vi "主程序-复材超声C扫缺陷分析评定软件.vi"() -> ()   [LabVIEW 2018]
doc: "使用该模板构建用户界面事件处理设计模式。将模板应用于对话框及其它用户界面。用户也可创建并执行VI可按照与用户界面事件相同方式处理的用户定义事件。"
uses:
  <vilib>/Utility/NIReport.llb/Report Type.ctl
  <vilib>/addons/_office/_exclsub.llb/font.ctl
  <vilib>/Utility/NIReport.llb/HTML Report Image Alignment.ctl
  <vilib>/Utility/NIReport.llb/Append Report Text (str wrap).vi
  <vilib>/Utility/NIReport.llb/Append Image to Report (path wrap).vi
  <vilib>/addons/_office/word.llb/Word Easy Table (str).vi
  <vilib>/Utility/NIReport.llb/NI_report.lvclass
  <vilib>/Utility/NIReport.llb/Word/NI_Word.lvclass
  <vilib>/addons/_office/NI_ReportGenerationToolkit.lvlib
  <vilib>/Utility/NIReport.llb/NI_ReportGenerationCore.lvlib
  <vilib>/vision/NI_Vision_Development_Module.lvlib
panel:
  out "是否需要预处理":u16
  out "数值":i8
  out "弥散类缺陷灰度阈值":dbl caption="值"
  out "计入分层缺陷的面积阈值":i32
  out "报告模式":string
  in  "删除标注":bool caption="定量分析"
  out "分层类缺陷灰度阈值":dbl caption="值"
  out "反射图原始路径":path
  out "穿透图原始路径":path
  out "ROImask":T1(plugin-control)
  out "模式选择":u16(ring) items=["只读穿透图", "穿透图和反射图结合"]
  out "添加的路径":path
  out "连接的字符串 2":string
  out "临界面积百分比值":dbl
  out "临界Z值":i32
  out "标注后的图片路径":path
  out "全部检测结果合并":string[][](table)
  out "全部检测结果":string[][](table)
  out "部位信息":string[](array[string])=["", "34.500000", "32.500000", "1121", "34", "54.955926", "分层类", "不合格", ""]
  out "连接的字符串":string
  in  "完成标注":bool caption="定量分析"
  out "框数":dbl
  out "自定义字体":T2={"Desired Font (Application)"=enum."Application Font", "[User-specified Font]"={"Font Name"="", "Size"=12, "Strikeout?"=FALSE, "Italic?"=FALSE, "Underline?"=FALSE, "Outline?"=FALSE, "Shadow?"=FALSE, "Bold?"=FALSE, "Rotation Angle"=0.0}, "Horizontal Alignment"=0, "Vertical Alignment"=0} {"Horizontal Alignment" items=["Left", "Center", "Right"]; "Vertical Alignment" items=["Bottom", "Top", "Baseline"]}
  out "框组":T3(array[cluster])
  out "质量等级":string
  in  "stop":bool caption="停止"
  in  "导入图像":bool caption="导入图片"
  in  "开始标注":bool caption="定量分析"
  in  "查看评定结果":bool caption="辅助定性分析"
  in  "生成报告":bool caption="生成原始记录"
  in  "控件":enum32{"穿透图", "反射图"}(tab)
  out "穿透图":T1(plugin-control)
  out "反射图":T1(plugin-control)
  out "产品规格":cluster{"产品长度（周长）（mm）":dbl, "产品宽度（母线长）（mm）":dbl}
  out "图像分辨率":T4
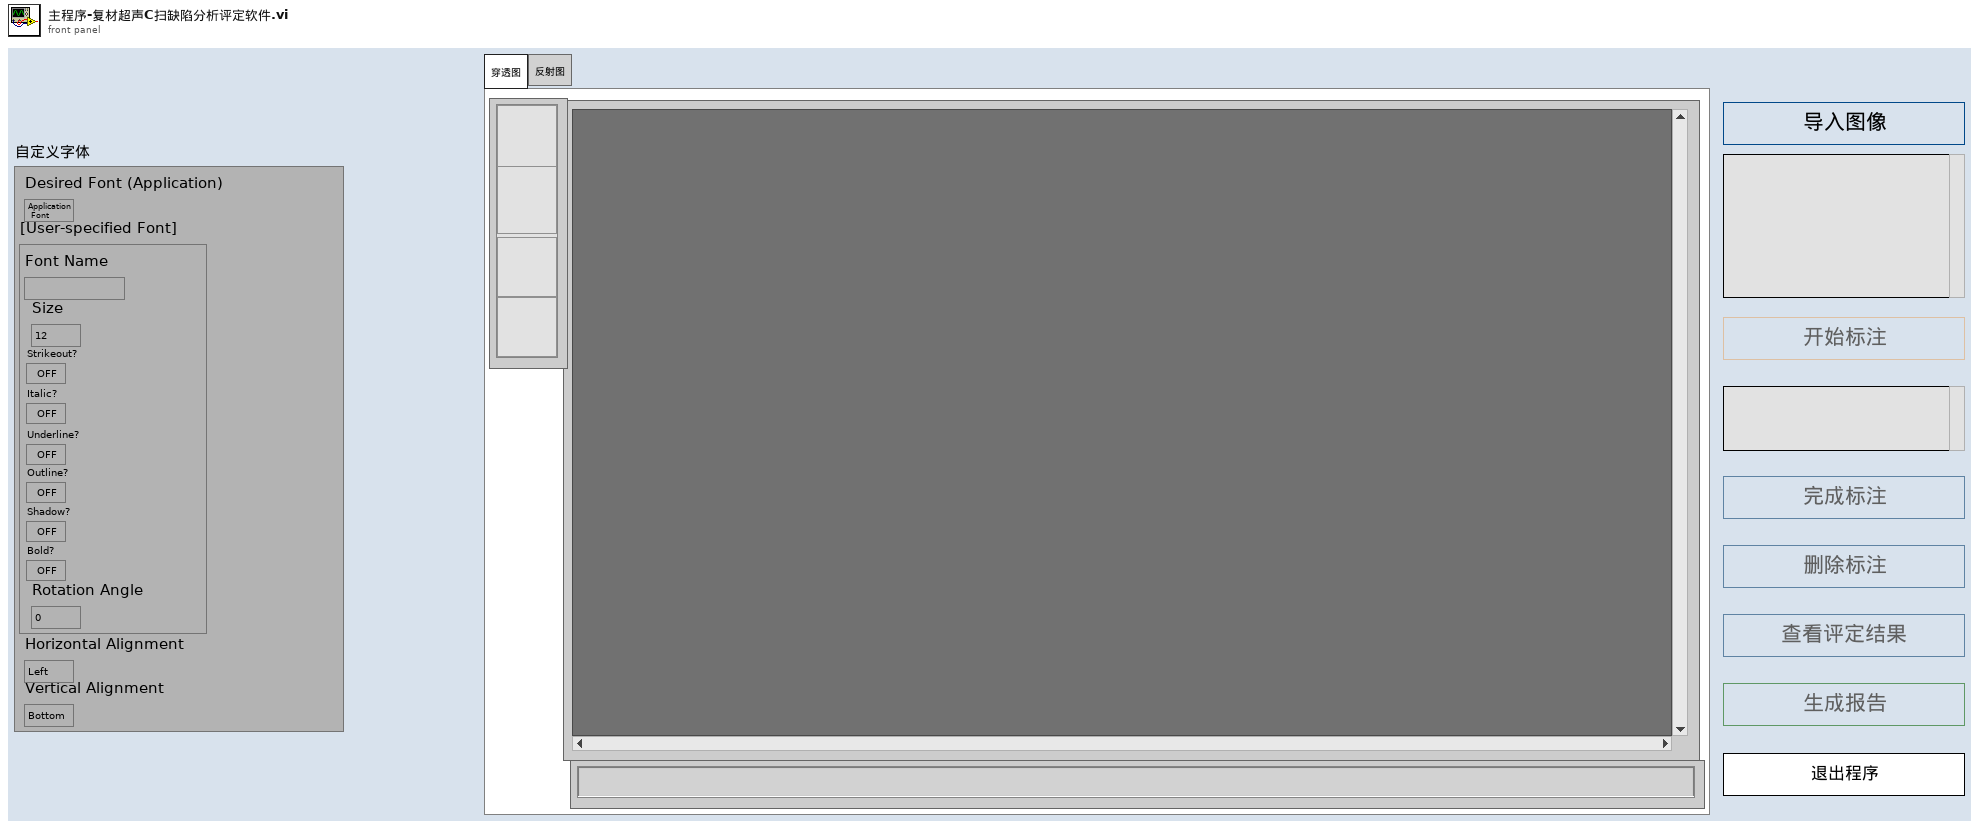
[diagram p1: front panel]
types:
  T1 = typedef "IMAQ Image.ctl" = refnum<image>
  T2 = cluster{"Desired Font (Application)":enum16{"User-specified Font", "Application Font", "System Font", "Dialog Font"}, "[User-specified Font]":cluster{"Font Name":string, "Size":i16, "Strikeout?":bool, "Italic?":bool, "Underline?":bool, "Outline?":bool, "Shadow?":bool, "Bold?":bool, "Rotation Angle":dbl}, "Horizontal Alignment":i16, "Vertical Alignment":i16}
  T3 = cluster{"Global Rectangle":i32[], "Contours":cluster{"Contour Type":u32, "ROI Type":u32, "Points":i32[]}[]}[]
  T4 = cluster{"图像X向分辨率（mm/像素）":dbl, "图像Y向分辨率（mm/像素）":dbl}
  T5 = enum8{"Enabled", "Disabled", "Disabled and Grayed Out"}
  T6 = cluster{"Global Rectangle":i32[], "Contours":cluster{"Contour Type":u32, "ROI Type":u32, "Points":i32[]}[]}
  T7 = cluster{"Zoom Tool":bool, "Selection Tool":bool, "Pan Tool":bool, "Point Tool":bool, "Line Tool":bool, "Rectangle Tool":bool, "Rotated Rectangle Tool":bool, "Polyline Tool":bool, "Polygon Tool":bool, "Freehand Tool":bool, "Closed Freehand Tool":bool, "Ellipse Tool":bool, "Annulus Tool":bool}
  T8 = enum16{"maximized", "minimized", "normal", "no change"}
  T9 = typedef "NI_ReportGenerationCore.lvlib/Report Type.ctl" = enum16{"HTML", "Word", "Excel"}
  T10 = typedef "NI_ReportGenerationCore.lvlib/HTML Report Image Alignment.ctl" = enum16{"(default)", "LEFT", "RIGHT", "TOP", "TEXTTOP", "MIDDLE", "ABSMIDDLE", "BASELINE", "BOTTOM", "ABSBOTTOM"}
  T11 = cluster{"position (Excel)":cluster{"row":i32, "column":i32}, "name (Excel)":string, "bookmark (Word)":string}
  T12 = cluster{"position (excel)":cluster{"row":i32, "column":i32}, "name (excel)":string, "bookmark (word)":string}
  T13 = typedef "NI_ReportGenerationToolkit.lvlib/font.ctl" = cluster{"font name":string, "font size":dbl, "bold":u16, "italic":u16, "underline":u16, "strike through":u16, "font color":u32}
  T14 = typedef "Image Type" = u32
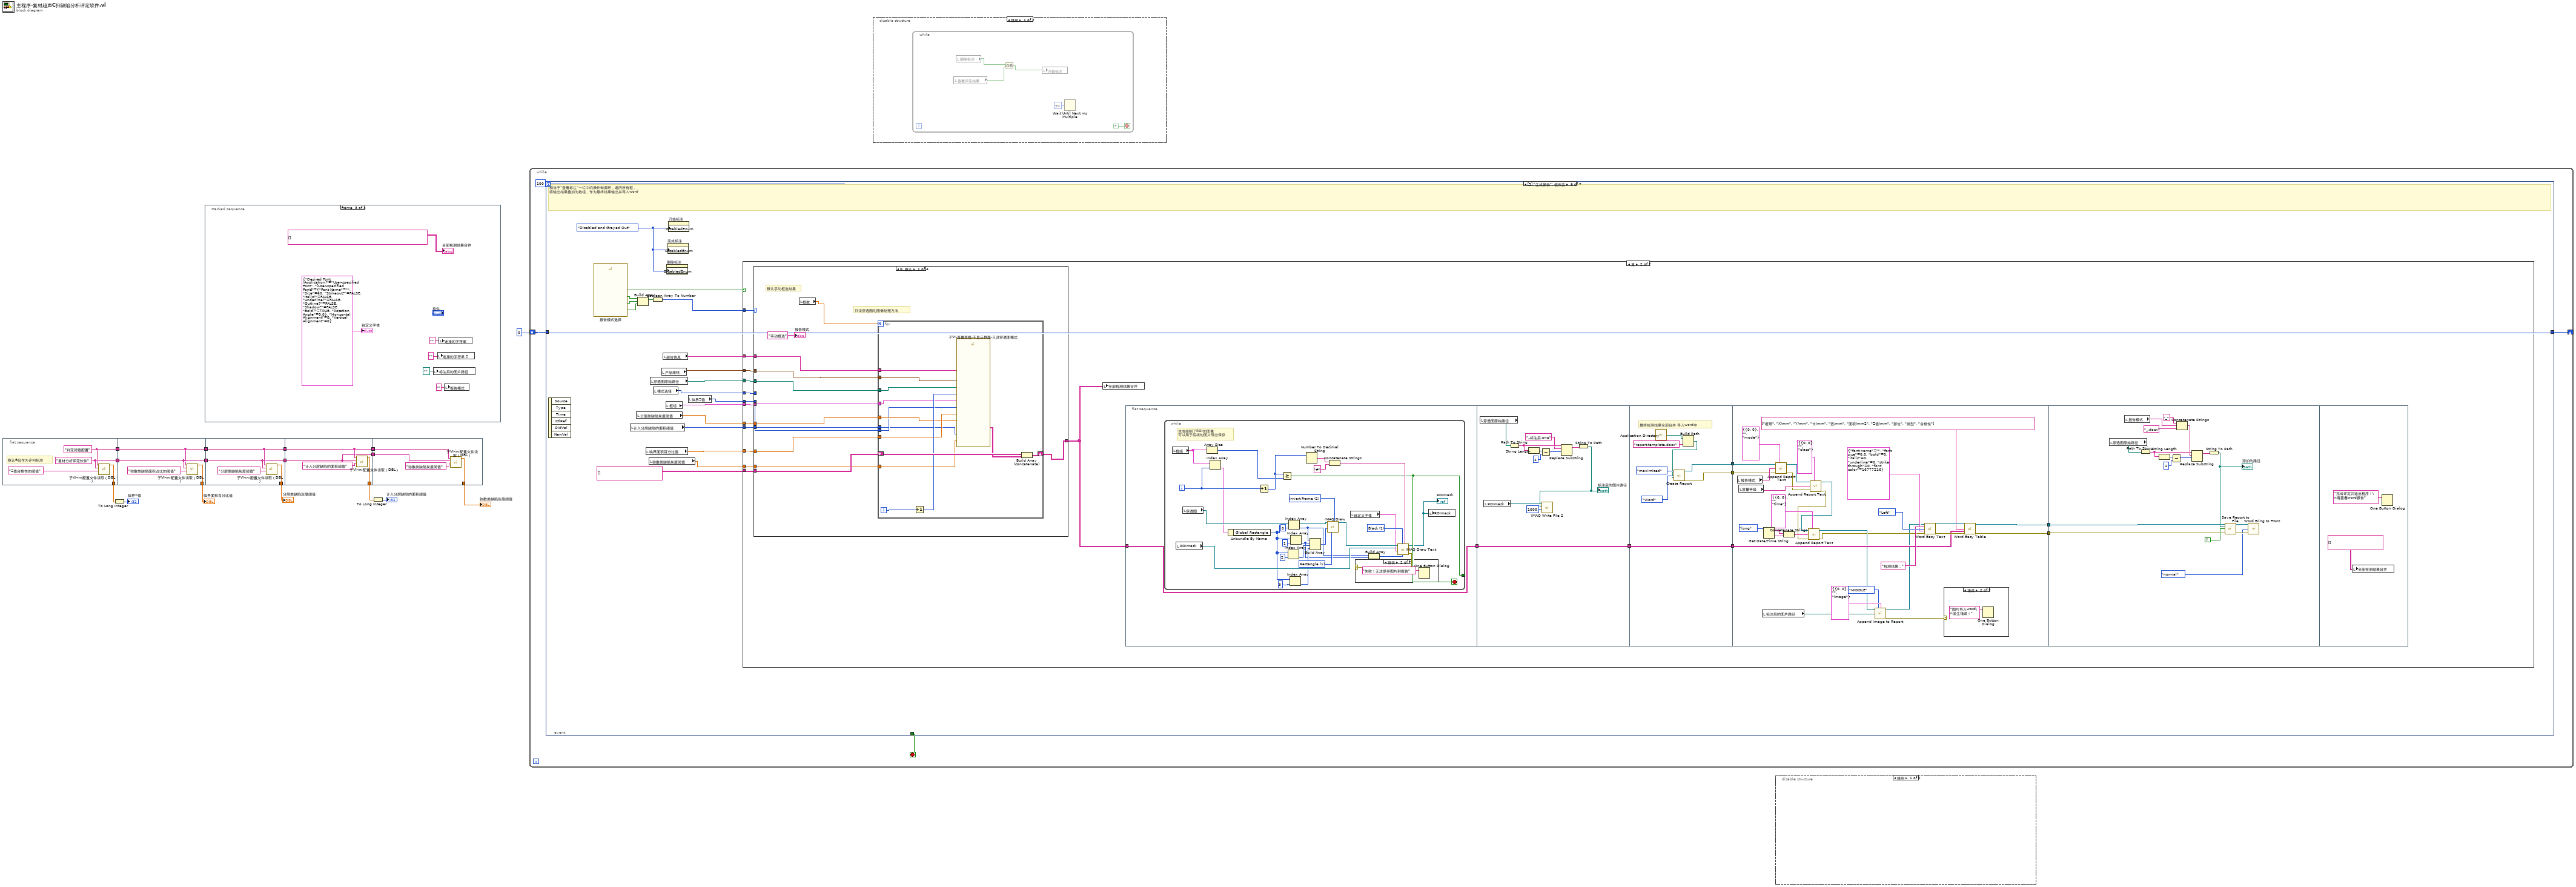
[diagram p0: block diagram]
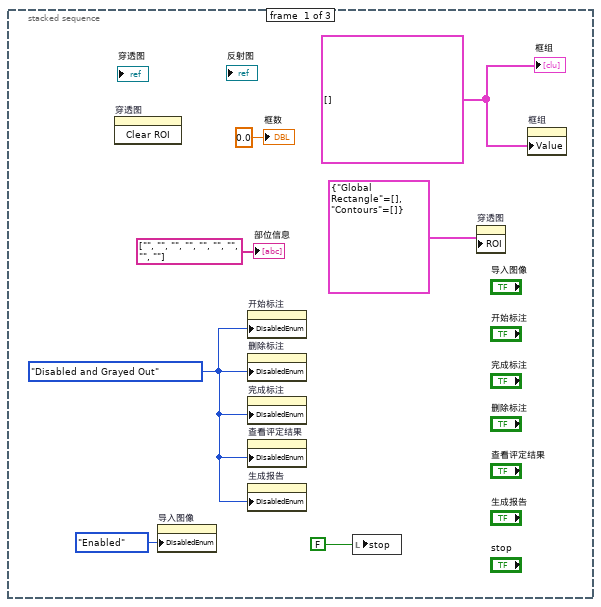
[diagram p3: hidden frame]
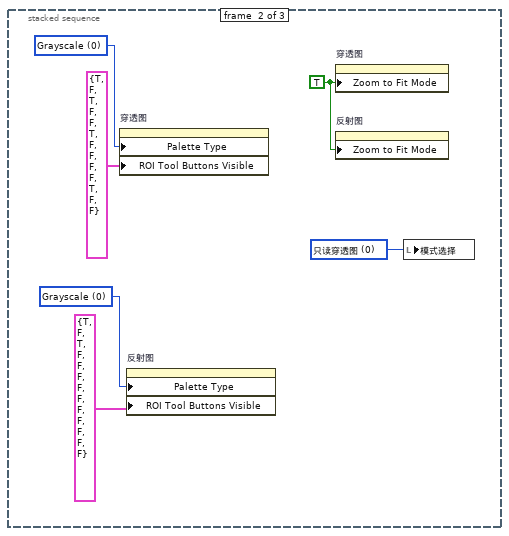
[diagram p4: hidden frame]
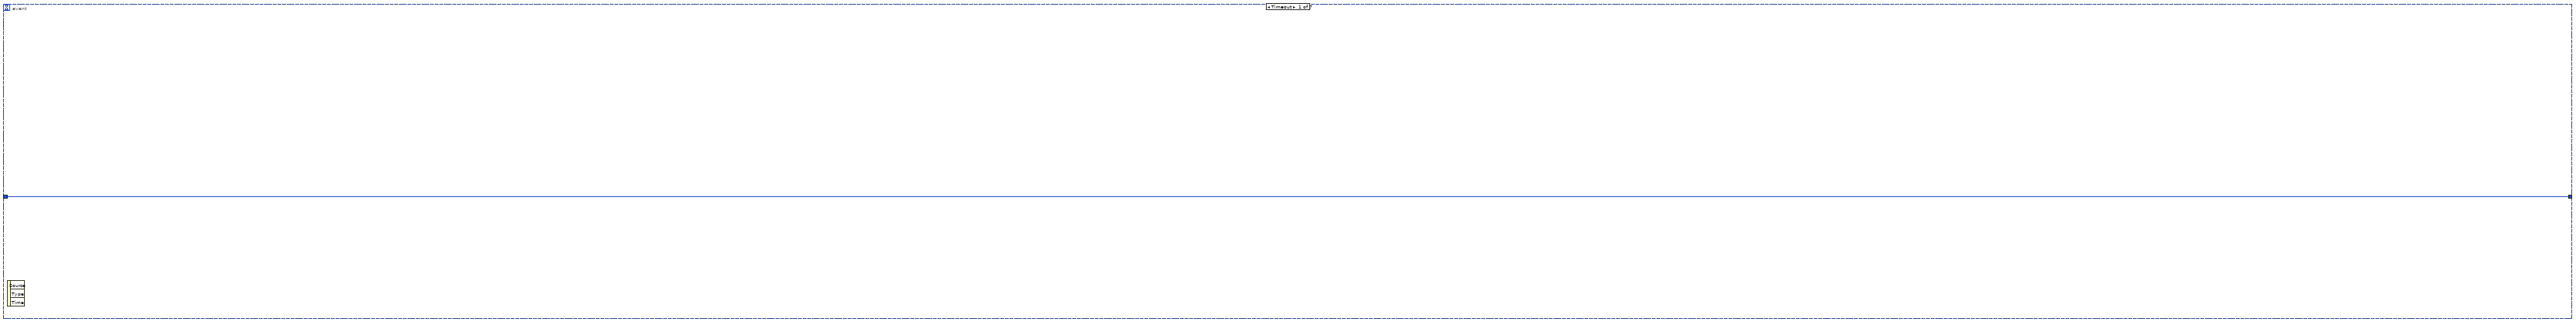
[diagram p6: hidden frame]
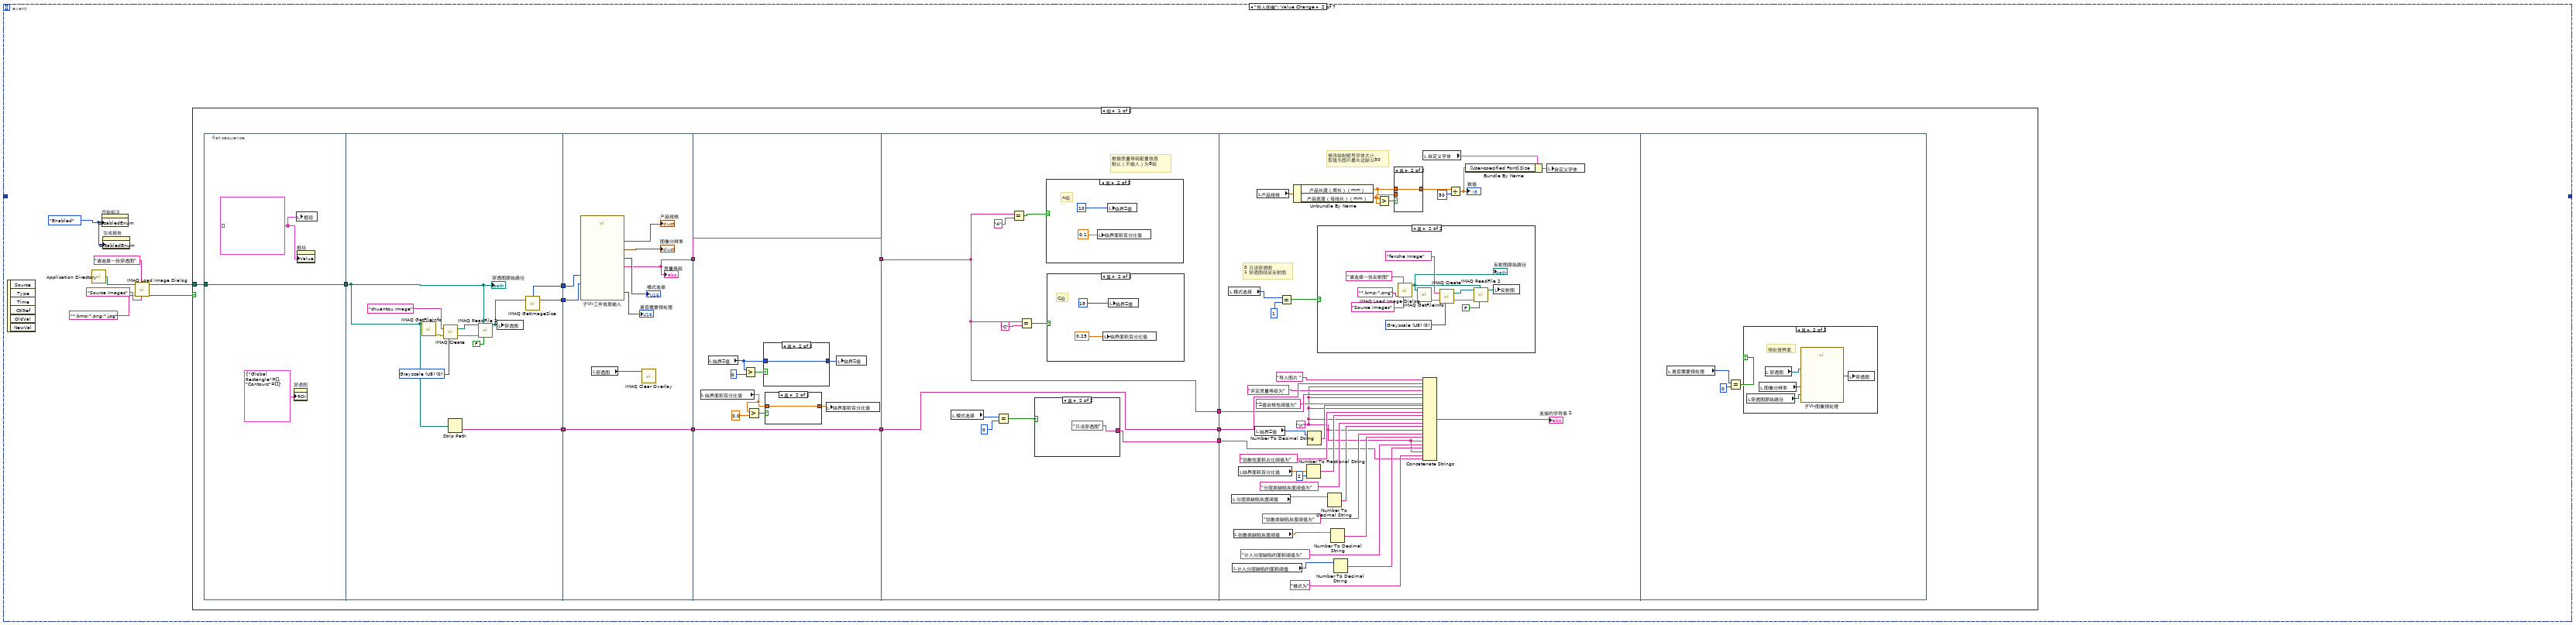
[diagram p7: hidden frame]
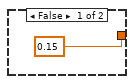
[diagram p8: hidden frame]
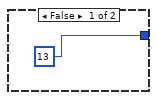
[diagram p9: hidden frame]
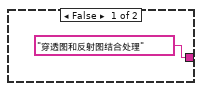
[diagram p10: hidden frame]
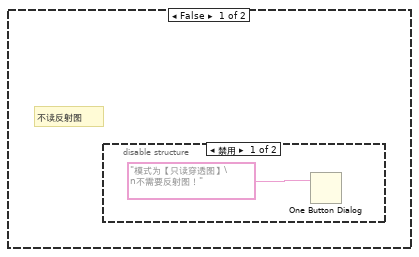
[diagram p14: hidden frame]
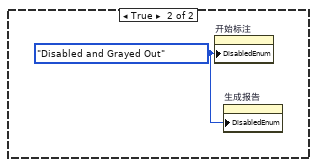
[diagram p17: hidden frame]
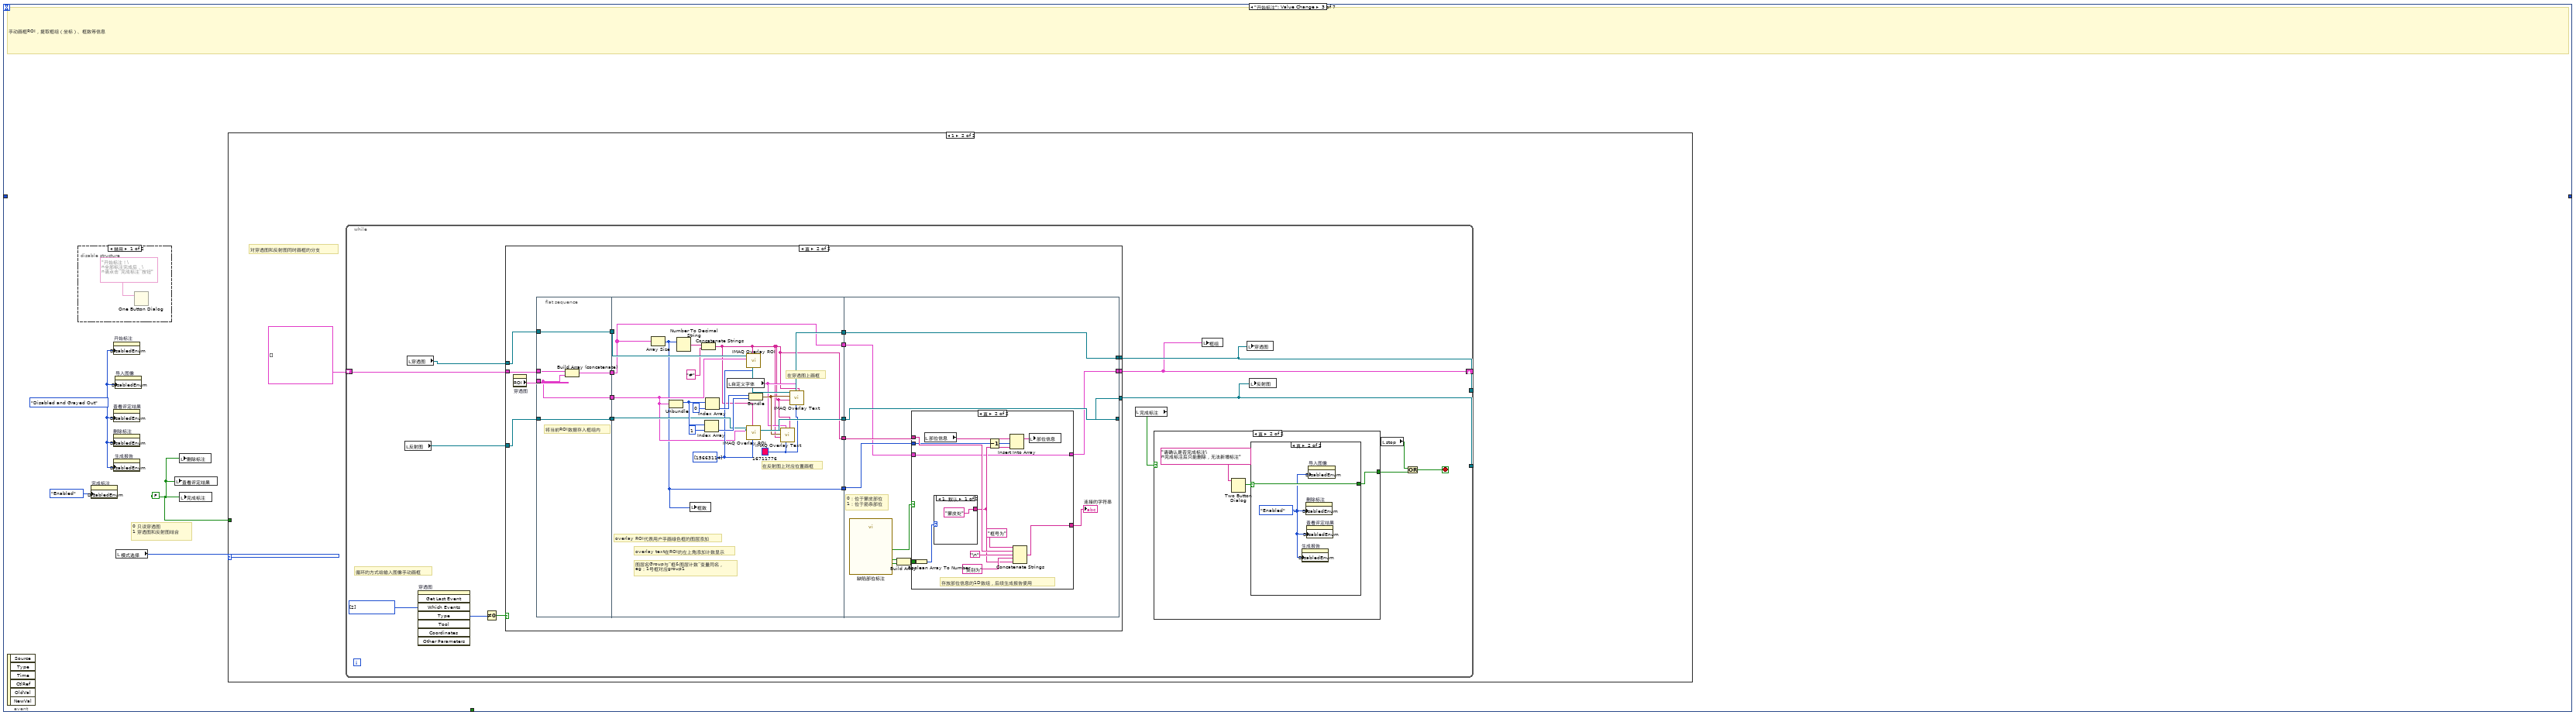
[diagram p18: hidden frame]
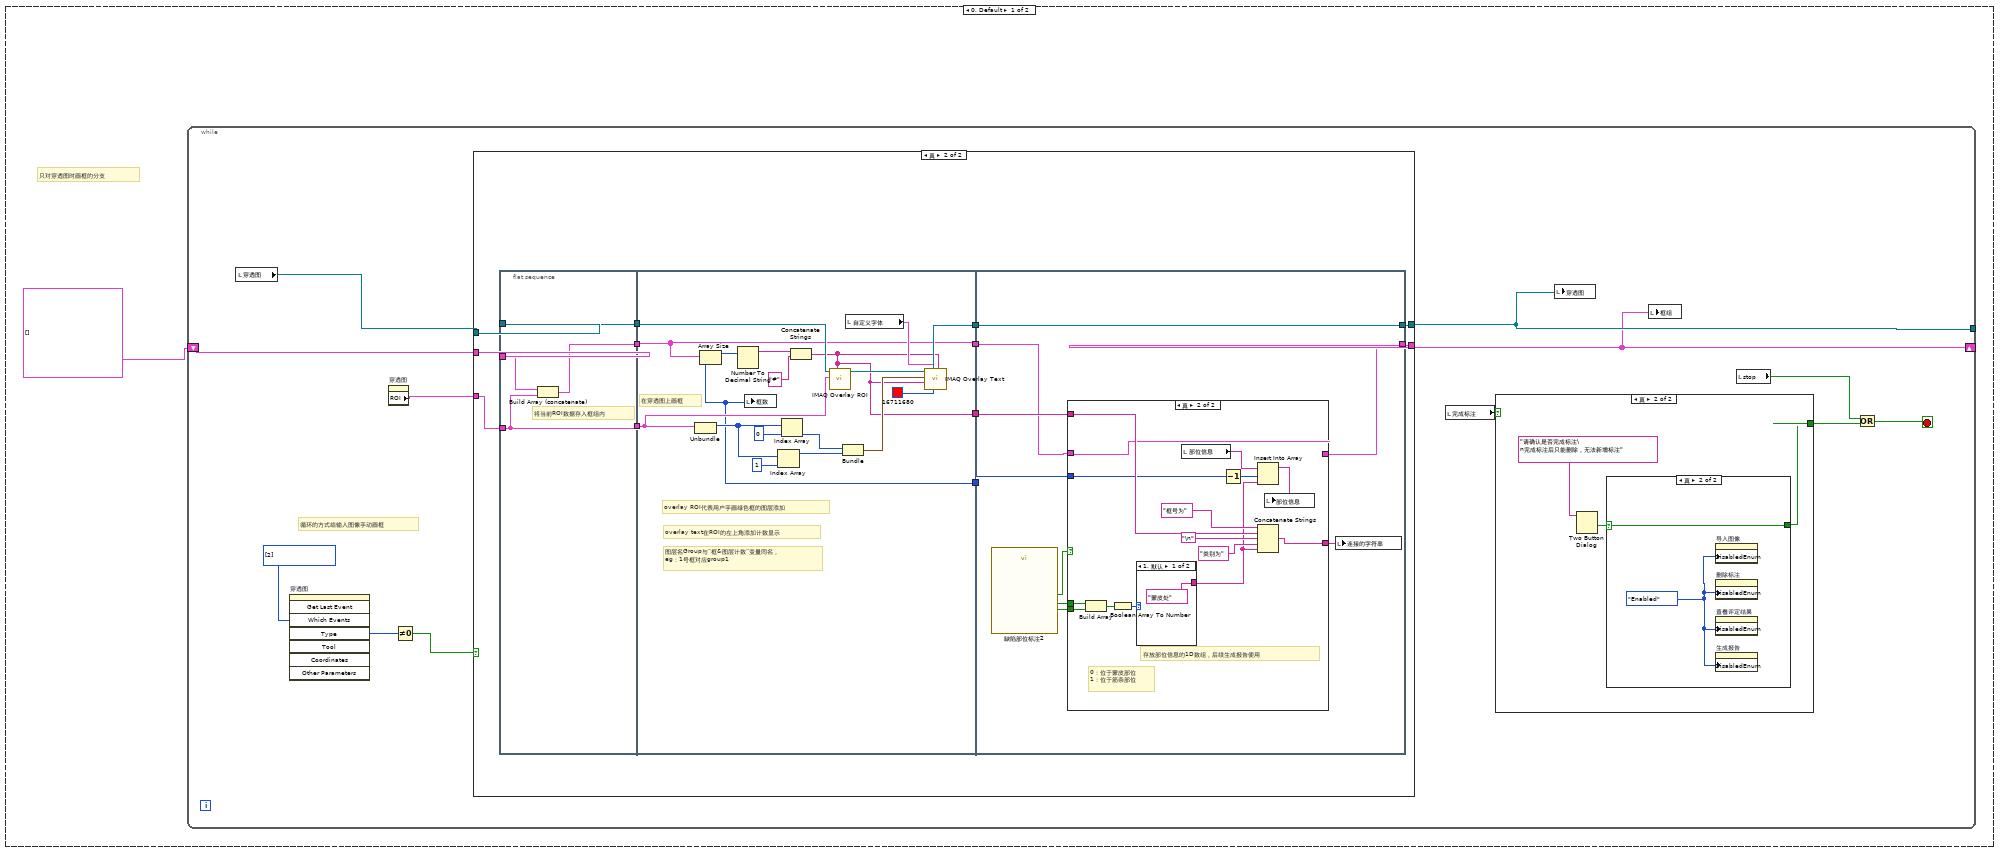
[diagram p20: hidden frame]
diagram:
  n1 = flat-sequence {
    tunnel: [w19] -> w15
    tunnel: [w18] -> w14
    tunnel: [w17] -> w9
    tunnel: w15 -> [w22]
    tunnel: w14 -> [w23]
    tunnel: [w23] -> w13
    tunnel: [w22] -> w12
    tunnel: [w21] -> w10
    tunnel: w13 -> [w25]
    tunnel: w12 -> [w26]
    tunnel: [w27] -> w11
    tunnel: [w26] -> w7
    tunnel: [w25] -> w6
    tunnel: w7 -> [w30]
    tunnel: w6 -> [w29]
    tunnel: [w31] -> w4
    tunnel: [w30] -> w3
    tunnel: [w29] -> w2
    tunnel: w3 -> [w35]
    tunnel: w2 -> [w34]
    tunnel: [w33] -> w1
    frame #0 {
      w18 = "复材分析评定软件" ("section")
      w19 = "判定阈值配置" ("文件名称")
      # "默认B级作为评判标准"
      n2 = call "子VI-ini配置文件读取（DBL）.vi"("key"="Z值合格性的阈值", "section"=w18, "文件名称"=w19) -> ("value"=w17:dbl)  [unwired: 8 in]
    }
    frame #1 {
      n3 = call "子VI-ini配置文件读取（DBL）.vi"("key"="弥散性缺陷面积占比的阈值", "section"=w23, "文件名称"=w22) -> ("value"=w21:dbl)  [unwired: 8 in]
    }
    frame #2 {
      n4 = call "子VI-ini配置文件读取（DBL）.vi"("key"="分层类缺陷灰度阈值", "section"=w25, "文件名称"=w26) -> ("value"=w27:dbl)  [unwired: 8 in]
    }
    frame #3 {
      n5 = call "子VI-ini配置文件读取（DBL）.vi"("key"="计入分层缺陷的面积阈值", "section"=w29, "文件名称"=w30) -> ("value"=w31:dbl)  [unwired: 8 in]
    }
    frame #4 {
      n6 = call "子VI-ini配置文件读取（DBL）.vi"("key"="弥散类缺陷灰度阈值", "section"=w34, "文件名称"=w35) -> ("value"=w33:dbl)  [unwired: 8 in]
    }
  }
  n7 = To Long Integer(number=w9) -> (32bit integer=→"临界Z值":i32)
  n8 = stacked-sequence {
    frame #0 {
      w41 = T3 [] ("框组")
      w38 = T5."Disabled and Grayed Out" ("禁用")
      n9 = invoke on="穿透图" class="ImageControl" method="Clear ROI"() -> ()  [unwired: 3 in, 3 out]
      n10 = property on="导入图像" class="Bool"("DisabledEnum"=T5."Enabled" ("禁用")) -> ()  [unwired: 2 in, 2 out]
      n11 = property on="开始标注" class="Bool"("DisabledEnum"=w38) -> ()  [unwired: 2 in, 2 out]
      n12 = property on="删除标注" class="Bool (严格)"("DisabledEnum"=w38) -> ()  [unwired: 2 in, 2 out]
      n13 = property on="完成标注" class="Bool (严格)"("DisabledEnum"=w38) -> ()  [unwired: 2 in, 2 out]
      n14 = property on="查看评定结果" class="Bool (严格)"("DisabledEnum"=w38) -> ()  [unwired: 2 in, 2 out]
      n15 = property on="生成报告" class="Bool"("DisabledEnum"=w38) -> ()  [unwired: 2 in, 2 out]
      n16 = local write "stop"(FALSE ("stop")) -> ()
      n17 = property on="穿透图" class="ImageControl"("ROI"=T6 {"Global Rectangle"=[], "Contours"=[]}) -> ()  [unwired: 2 in, 2 out]
      n18 = property on="框组" class="Arr (严格)"("Value"=w41) -> ()  [unwired: 2 in, 2 out]
      "部位信息" <- string[] ["", "", "", "", "", "", "", "", ""] ("部位信息")
      "框组" <- w41
      "框数" <- 0.0 ("框数")
    }
    frame #1 {
      w44 = u16 0 items=["只读穿透图", "穿透图和反射图结合"] ("模式选择")
      w46 = u32 0 items=["Grayscale", "Binary", "Gradient", "Rainbow", "Temperature", "User Defined", "Binary 16 Bit", "Gradient 16 Bit", "Rainbow 16 Bit", "Temperature 16 Bit", "User Defined 16 Bit"] ("Palette:Palette Type")
      w47 = TRUE ("Zoom to Fit Mode")
      w49 = u32 0 items=["Grayscale", "Binary", "Gradient", "Rainbow", "Temperature", "User Defined", "Binary 16 Bit", "Gradient 16 Bit", "Rainbow 16 Bit", "Temperature 16 Bit", "User Defined 16 Bit"] ("Palette:Palette Type")
      n19 = property on="穿透图" class="ImageControl"("Palette Type"=w49, "ROI Tool Buttons Visible"=T7 {"Zoom Tool"=TRUE, "Selection Tool"=FALSE, "Pan Tool"=TRUE, "Point Tool"=FALSE, "Line Tool"=FALSE, "Rectangle Tool"=TRUE, "Rotated Rectangle Tool"=FALSE, "Polyline Tool"=FALSE, "Polygon Tool"=FALSE, "Freehand Tool"=FALSE, "Closed Freehand Tool"=TRUE, "Ellipse Tool"=FALSE, "Annulus Tool"=FALSE} ("ROI Tool Buttons Visible:All Elements")) -> ()  [unwired: 2 in, 2 out]
      n20 = property on="反射图" class="ImageControl"("Palette Type"=w46, "ROI Tool Buttons Visible"=T7 {"Zoom Tool"=TRUE, "Selection Tool"=FALSE, "Pan Tool"=TRUE, "Point Tool"=FALSE, "Line Tool"=FALSE, "Rectangle Tool"=FALSE, "Rotated Rectangle Tool"=FALSE, "Polyline Tool"=FALSE, "Polygon Tool"=FALSE, "Freehand Tool"=FALSE, "Closed Freehand Tool"=FALSE, "Ellipse Tool"=FALSE, "Annulus Tool"=FALSE} ("ROI Tool Buttons Visible:All Elements")) -> ()  [unwired: 2 in, 2 out]
      n21 = property on="穿透图" class="ImageControl"("Zoom to Fit Mode"=w47) -> ()  [unwired: 2 in, 2 out]
      n22 = property on="反射图" class="ImageControl"("Zoom to Fit Mode"=w47) -> ()  [unwired: 2 in, 2 out]
      n23 = local write "模式选择"(w44) -> ()
    }
    frame #2 {
      n24 = local write "标注后的图片路径"(path "" ("标注后的图片路径")) -> ()
      n25 = local write "连接的字符串 2"("" ("连接的字符串 2")) -> ()
      n26 = local write "连接的字符串"("" ("连接的字符串")) -> ()
      n27 = local write "报告模式"("" ("报告模式")) -> ()
      "自定义字体" <- T2 {"Desired Font (Application)"=enum."User-specified Font", "[User-specified Font]"={"Font Name"="", "Size"=60, "Strikeout?"=FALSE, "Italic?"=FALSE, "Underline?"=FALSE, "Outline?"=FALSE, "Shadow?"=FALSE, "Bold?"=TRUE, "Rotation Angle"=0.0}, "Horizontal Alignment"=0, "Vertical Alignment"=0} ("Font, Size & Style")
      "全部检测结果合并" <- string[][] [] ("弥散类检测结果合并")
    }
  }
  n28 = To Long Integer(number=w4) -> (32bit integer=→"计入分层缺陷的面积阈值":i32)
  n29 = while {
    shift-right: [w56] -> _
    shift-left: 0 -> [w57]
    stop <- w59 stop-if-true
    n30 = event shown="[5] \"生成报告\": 值改变" {
      selector: _ -> [_ _ _ _ _ _ _]
      dyn-events: _ -> [_ _ _ _ _ _ _]
      timeout: 100 -> [_ _ _ _ _ _ _]
      tunnel: [_ _ _ _ _ _ w643] -> w59
      tunnel: w57 -> [w60 _ _ _ _ w440 _]
      tunnel: [w60 _ _ _ _ w440 0] -> w56
      event Timeout {
        n31 = event-data() -> ()  [unwired: 1 in, 3 out]
      }
      event "导入图像": Value Change {
        w62 = T5."Enabled" ("禁用")
        n32 = event-data() -> ()  [unwired: 1 in, 6 out]
        n33 = call <vilib>:"Application Directory.vi"() -> ("Application Directory"=w61:path)
        n34 = property on="开始标注" class="Bool"("DisabledEnum"=w62) -> ()  [unwired: 2 in, 2 out]
        n35 = property on="生成报告" class="Bool"("DisabledEnum"=w62) -> ()  [unwired: 2 in, 2 out]
        n36 = call "IMAQ Load Image Dialog"("Pattern Label"="Source Images", "Prompt"="请选择一张穿透图" ("prompt"), "Pattern"="*.bmp;*.png;*.jpg", "Start Path"=w61) -> ("Cancelled?"=w64:bool, "Path"=w63:path)  [unwired: 5 in, 1 out]
        n37 = case shown="假" w64 {
          tunnel: w63 -> [w77 _]
          frame False {
            n38 = flat-sequence {
              tunnel: w77 -> [w80]
              tunnel: [w80] -> w76
              tunnel: w76 -> [w84]
              tunnel: [w86] -> w75
              tunnel: [w85] -> w74
              tunnel: [w83] -> w73
              tunnel: [w99] -> w79
              tunnel: w75 -> [w98]
              tunnel: w74 -> [w97]
              tunnel: w73 -> [w96]
              tunnel: [w96] -> w72
              tunnel: w79 -> [w112]
              tunnel: [w112] -> w78
              tunnel: w72 -> [w111]
              tunnel: [w111] -> w71
              tunnel: w78 -> [w118]
              tunnel: w71 -> [w119]
              tunnel: [w119] -> w70
              tunnel: [w118] -> w69
              tunnel: [w117] -> w68
              tunnel: w70 -> [w156]
              tunnel: w69 -> [w154]
              tunnel: w68 -> [w142]
              frame #0 {
                w81 = T3 [] ("框组")
                n39 = property on="穿透图" class="ImageControl"("ROI"=T6 {"Global Rectangle"=[], "Contours"=[]}) -> ()  [unwired: 2 in, 2 out]
                n40 = local write "框组"(w81) -> ()
                n41 = property on="框组" class="Arr (严格)"("Value"=w81) -> ()  [unwired: 2 in, 2 out]
              }
              frame #1 {
                w88 = T14 0 items=["Grayscale (U8)", "Grayscale (I16)", "Grayscale (SGL)", "Complex (CSG)", "RGB (U32)", "HSL (U32)", "RGB (U64)", "Grayscale (U16)"] ("Image Type")
                n42 = call "IMAQ GetFileInfo"("File Path"=w84) -> ("error out"=w91:errorcluster)  [unwired: 4 in, 6 out]
                n43 = call "IMAQ Create"("Image Name"="chuantou Image", "Image Type"=w88, "error in (no error)"=w91) -> ("New Image"=w92:T1, "error out"=w93:errorcluster)  [unwired: 2 in]
                n44 = Strip Path(path=w84) -> (name=w83:string)  [unwired: 1 out]
                n45 = call "IMAQ ReadFile 2"("Use File Path Image Type"=FALSE, "File Path"=w84, "error in (no error)"=w93, "Image"=w92) -> ("Image Out"=w90:T1)  [unwired: 3 in, 4 out]
                n46 = local write "穿透图"(w90) -> ()
                n47 = call "IMAQ GetImageSize"("Image"=w90) -> ("Y Resolution"=w85:i32, "X Resolution"=w86:i32)  [unwired: 3 in, 1 out]
                "穿透图原始路径" <- w84
              }
              frame #2 {
                n48 = call "子VI-工件信息输入.vi"("Y Resolution"=w97, "X Resolution"=w98) -> ("质量等级"=w99:string, "模式选择"=→"模式选择":u16, "产品规格"=→"产品规格":cluster{"产品长度（周长）（mm）":dbl, "产品宽度（母线长）（mm）":dbl}, "是否需要预处理"=→"是否需要预处理":u16, "图像分辨率"=→"图像分辨率":T4)  [unwired: 5 in]
                "质量等级" <- w99
                n49 = local read "穿透图"() -> (w95:T1)
                n50 = call "IMAQ Clear Overlay"("Image"=w95) -> ()  [unwired: 9 in, 2 out]
              }
              frame #3 {
                n51 = local read "临界面积百分比值"() -> (w103:dbl)
                n52 = local read "临界Z值"() -> (w104:i32)
                n53 = Greater?(x=w104, y=0) -> (0:w109:bool)
                n54 = Greater?(x=w103, y=0.0) -> (0:w107:bool)
                n55 = case shown="真" w109 {
                  tunnel: [13 ("临界Z值") w116] -> w106
                  tunnel: w104 -> [_ w116]
                  frame False {
                  }
                  frame True {
                  }
                }
                n56 = case shown="真" w107 {
                  tunnel: [0.15 ("临界面积百分比值") w114] -> w105
                  tunnel: w103 -> [_ w114]
                  frame False {
                  }
                  frame True {
                  }
                }
                n57 = local write "临界面积百分比值"(w105) -> ()
                n58 = local write "临界Z值"(w106) -> ()
              }
              frame #4 {
                # "根据质量等级配置信息\n默认（不输入）为B级"
                n59 = local read "模式选择"() -> (w121:u16)
                n60 = Equal?(x=w121, y=u16 0) -> (x = y?=w120:bool)
                n61 = Equal?(x=w118, y="A") -> (x = y?=w125:bool)
                n62 = Equal?(x=w118, y="C") -> (x = y?=w126:bool)
                n63 = case shown="真" w120 {
                  tunnel: ["穿透图和反射图结合处理" ("字符串") "只读穿透图" ("字符串")] -> w117
                  frame False {
                  }
                  frame True {
                  }
                }
                n64 = case shown="真" w125 {
                  frame False {
                  }
                  frame True {
                    # "A级"
                    n65 = local write "临界面积百分比值"(0.1 ("临界面积百分比值")) -> ()
                    n66 = local write "临界Z值"(10 ("临界Z值")) -> ()
                  }
                }
                n67 = case shown="真" w126 {
                  frame False {
                  }
                  frame True {
                    # "C级"
                    n68 = local write "临界面积百分比值"(0.25 ("临界面积百分比值")) -> ()
                    n69 = local write "临界Z值"(19 ("临界Z值")) -> ()
                  }
                }
              }
              frame #5 {
                w144 = "\n"
                # "修改绘制框号字体大小\n取值为图片最长边除以50"
                # "0 只读穿透图\n1 穿透图结合反射图"
                n70 = local read "模式选择"() -> (w167:u16)
                n71 = local read "分层类缺陷灰度阈值"() -> (w164:dbl)
                n72 = local read "计入分层缺陷的面积阈值"() -> (w147:i32)
                n73 = local read "弥散类缺陷灰度阈值"() -> (w150:dbl)
                n74 = local read "临界面积百分比值"() -> (w162:dbl)
                n75 = local read "临界Z值"() -> (w160:i32)
                n76 = local read "产品规格"() -> (w134:cluster{"产品长度（周长）（mm）":dbl, "产品宽度（母线长）（mm）":dbl})
                n77 = Equal?(x=w167, y=u16 1) -> (x = y?=w166:bool)
                n78 = Unbundle By Name(w134) -> ("产品长度（周长）（mm）"=w136:dbl, "产品宽度（母线长）（mm）"=w137:dbl)
                n79 = Number To Fractional String(number=w162, precision (6)=i16 2 ("精度(6)")) -> (F-format string=w163:string)  [unwired: 2 in]
                n80 = Number To Decimal String(number=w160) -> (decimal integer string=w161:string)  [unwired: 1 in]
                n81 = case shown="真" w166 {
                  frame False {
                    # "不读反射图"
                    n82 = disable-structure shown="禁用" {
                      frame Disabled {
                        n83 = One Button Dialog(message="模式为【只读穿透图】\n不需要反射图！" ("消息")) -> ()  [unwired: 1 in, 1 out]
                      }
                      frame Enabled {
                      }
                    }
                  }
                  frame True {
                    w174 = T14 0 items=["Grayscale (U8)", "Grayscale (I16)", "Grayscale (SGL)", "Complex (CSG)", "RGB (U32)", "HSL (U32)", "RGB (U64)", "Grayscale (U16)"] ("Image Type")
                    n84 = call "IMAQ Load Image Dialog"("Pattern Label"="Source Images", "Prompt"="请选择一张反射图" ("prompt"), "Pattern"="*.bmp;*.png") -> ("Path"=w173:path)  [unwired: 6 in, 2 out]
                    "反射图原始路径" <- w173
                    n85 = call "IMAQ GetFileInfo"("File Path"=w173) -> ("error out"=w177:errorcluster)  [unwired: 4 in, 6 out]
                    n86 = call "IMAQ Create"("Image Name"="fanshe Image", "Image Type"=w174, "error in (no error)"=w177) -> ("New Image"=w178:T1, "error out"=w179:errorcluster)  [unwired: 2 in]
                    n87 = call "IMAQ ReadFile 2"("Use File Path Image Type"=FALSE, "File Path"=w173, "error in (no error)"=w179, "Image"=w178) -> ("Image Out"=w172:T1)  [unwired: 3 in, 4 out]
                    n88 = local write "反射图"(w172) -> ()
                  }
                }
                n89 = Number To Decimal String(number=w164) -> (decimal integer string=w165:string)  [unwired: 1 in]
                n90 = Number To Decimal String(number=w150) -> (decimal integer string=w148:string)  [unwired: 1 in]
                n91 = Number To Decimal String(number=w147) -> (decimal integer string=w145:string)  [unwired: 1 in]
                n92 = Greater?(x=w136, y=w137) -> (0:w135:bool)
                n93 = case shown="真" w135 {
                  tunnel: w136 -> [_ w170]
                  tunnel: w137 -> [w169 _]
                  tunnel: [w169 w170] -> w140
                  frame False {
                  }
                  frame True {
                  }
                }
                n94 = local read "自定义字体"() -> (w138:T2)
                n95 = Concatenate Strings("导入图片 " ("字符串"), w156, w144, "评定质量等级为" ("字符串"), w154, w144, "Z值合格性阈值为" ("字符串"), w161, w144, "弥散性面积占比阈值为" ("字符串"), w163, w144, "分层类缺陷灰度阈值为" ("字符串"), w165, w144, "弥散类缺陷灰度阈值为" ("字符串"), w148, w144, "计入分层缺陷的面积阈值为" ("字符串"), w145, w144, "模式为" ("字符串"), w142) -> (→"连接的字符串 2":string)
                n96 = Divide(x=w140, y=i8 50) -> (x/y=w141:dbl)
                "数值" <- w141
                n97 = Bundle By Name(cluster=w138, "[User-specified Font].Size"=w141) -> (w139:T2)
                n98 = local write "自定义字体"(w139) -> ()
              }
              frame #6 {
                n99 = local read "是否需要预处理"() -> (w184:u16)
                n100 = Equal?(x=w184, y=u16 0) -> (x = y?=w185:bool)
                n101 = case shown="真" w185 {
                  frame False {
                  }
                  frame True {
                    # "预处理界面"
                    n102 = local read "穿透图原始路径"() -> (w186:path)
                    n103 = local read "图像分辨率"() -> (w187:T4)
                    n104 = local read "穿透图"() -> (w189:T1)
                    n105 = call "子VI-图像预处理.vi"("图像分辨率"=w187, "穿透图"=w189, "穿透图原始路径"=w186) -> ("穿透图out"=w188:T1)  [unwired: 8 in]
                    n106 = local write "穿透图"(w188) -> ()
                  }
                }
              }
            }
          }
          frame True {
            w190 = T5."Disabled and Grayed Out" ("禁用")
            n107 = property on="开始标注" class="Bool"("DisabledEnum"=w190) -> ()  [unwired: 2 in, 2 out]
            n108 = property on="生成报告" class="Bool"("DisabledEnum"=w190) -> ()  [unwired: 2 in, 2 out]
          }
        }
      }
      event "开始标注": Value Change {
        w191 = T5."Disabled and Grayed Out" ("禁用")
        w193 = FALSE ("完成标注")
        # "0 只读穿透图\n1 穿透图和反射图结合"
        # "手动画框ROI，提取框组（坐标）、框数等信息"
        n109 = event-data() -> ()  [unwired: 1 in, 6 out]
        n110 = disable-structure shown="禁用" {
          frame Disabled {
            n111 = One Button Dialog(message="开始标注！\n全部标注完成后，\n请点击“完成标注”按钮" ("消息")) -> ()  [unwired: 1 in, 1 out]
          }
          frame Enabled {
          }
        }
        n112 = property on="完成标注" class="Bool (严格)"("DisabledEnum"=T5."Enabled" ("禁用")) -> ()  [unwired: 2 in, 2 out]
        n113 = property on="查看评定结果" class="Bool (严格)"("DisabledEnum"=w191) -> ()  [unwired: 2 in, 2 out]
        n114 = property on="删除标注" class="Bool (严格)"("DisabledEnum"=w191) -> ()  [unwired: 2 in, 2 out]
        n115 = property on="生成报告" class="Bool"("DisabledEnum"=w191) -> ()  [unwired: 2 in, 2 out]
        n116 = property on="开始标注" class="Bool"("DisabledEnum"=w191) -> ()  [unwired: 2 in, 2 out]
        n117 = property on="导入图像" class="Bool"("DisabledEnum"=w191) -> ()  [unwired: 2 in, 2 out]
        n118 = local read "模式选择"() -> (w194:u16)
        n119 = local write "查看评定结果"(w193) -> ()
        n120 = local write "删除标注"(w193) -> ()
        n121 = local write "完成标注"(w193) -> ()
        n122 = case shown="1" w194 {
          tunnel: w193 -> [_ _]
          frame 0, Default {
            # "只对穿透图时画框的分支"
            n123 = while {
              shift-right: [w198] -> _
              shift-left: T3 [] ("框组") -> [w208]
              tunnel: [w206] -> _
              stop <- w197 stop-if-true
              (unwired) "_" ("名称或相对路径")
              (unwired) ".docx" ("名称或相对路径")
              w204 = i32[] [2] items=["No Event"=0, "Click Event"=1, "Draw Event"=2, "Size Event"=4, "Scroll Event"=5, "Double Click Event"=8] ("Which Events")
              # "循环的方式给输入图像手动画框"
              n124 = local read "穿透图"() -> (w207:T1)
              n125 = invoke on="穿透图" class="ImageControl" method="Get Last Event"("Which Events"=w204) -> ("Type"=w200:i32)  [unwired: 7 in, 7 out]
              n126 = property on="穿透图" class="ImageControl"() -> ("ROI"=w202:T6)  [unwired: 2 in, 2 out]
              n127 = Not Equal To 0?(x=w200) -> (x != 0?=w199:bool)
              n128 = case shown="真" w199 {
                tunnel: w207 -> [w219 w231]
                tunnel: [w219 w230] -> w206
                tunnel: [w217 w228] -> w198
                tunnel: w208 -> [w217 w229]
                tunnel: w202 -> [_ w227]
                frame False {
                  n129 = Wait (ms)(milliseconds to wait=u32 50 ("毫秒倍数")) -> ()  [unwired: 1 out]
                  n130 = Wait (ms)(milliseconds to wait=u32 50) -> ()  [unwired: 1 out]
                }
                frame True {
                  n131 = flat-sequence {
                    tunnel: w231 -> [w232]
                    tunnel: [w232] -> w226
                    tunnel: w227 -> [w235]
                    tunnel: [w235] -> w225
                    tunnel: w229 -> [w234]
                    tunnel: [w233] -> w224
                    tunnel: w226 -> [w244]
                    tunnel: w225 -> [w243]
                    tunnel: w224 -> [w236]
                    tunnel: [w246] -> w223
                    tunnel: [w236] -> w222
                    tunnel: [w240] -> w221
                    tunnel: [w238] -> w220
                    tunnel: w223 -> [w261]
                    tunnel: w222 -> [w255]
                    tunnel: w221 -> [w258]
                    tunnel: w220 -> [w257]
                    tunnel: [w261] -> w230
                    tunnel: [w254] -> w228
                    frame #0 {
                      # "将当前ROI数据存入框组内"
                      n132 = Build Array (concatenate)(w234, w235) -> (w233:T3)
                    }
                    frame #1 {
                      # "在穿透图上画框"
                      # "图层名Group与“框&图层计数”变量同名，\neg：1号框对应group1"
                      # "overlay text在ROI的左上角添加计数显示"
                      # "overlay ROI代表用户手画绿色框的图层添加"
                      n133 = Unbundle(w243) -> ("Global Rectangle"=w251:i32[])  [unwired: 1 out]
                      n134 = Array Size(array=w236) -> (size(s)=w238:i32)
                      n135 = Number To Decimal String(number=w238) -> (decimal integer string=w239:string)  [unwired: 1 in]
                      n136 = local write "框数"(w238) -> ()
                      n137 = Index Array(array=w251, index=1 ("索引")) -> (element=w249:i32)
                      n138 = Index Array(array=w251, index=0 ("索引")) -> (element=w250:i32)
                      n139 = Concatenate Strings(w239, "#" ("字符串")) -> (w240:string)
                      n140 = call "IMAQ Overlay ROI"("Group"=w240, "ROI Descriptor"=w243, "Image"=w244) -> ("Image Out"=w252:T1)  [unwired: 7 in, 1 out]
                      n141 = Bundle(w250, w249) -> (w245:cluster{i32, i32})  [unwired: 1 in]
                      n142 = local read "自定义字体"() -> (w242:T2)
                      n143 = call "IMAQ Overlay Text"("Group"=w240, "Text Color (black)"=u32 16711680, "Font, Size & Style"=w242, "String"=w240, "Origin"=w245, "Image"=w252) -> ("Image Out"=w246:T1)  [unwired: 4 in, 1 out]
                    }
                    frame #2 {
                      n144 = call "缺陷部位标注2"() -> ("位于筋条处"=w260:bool, "位于蒙皮处"=w259:bool, "确定"=w256:bool)  [unwired: 16 in, 1 out]
                      n145 = case shown="真" w256 {
                        tunnel: w260 -> [_ w277]
                        tunnel: w259 -> [_ w276]
                        tunnel: w258 -> [_ w272]
                        tunnel: w257 -> [_ w269]
                        tunnel: w255 -> [w264 w266]
                        tunnel: [w263 w266] -> w254
                        tunnel: ["由于点击取消，该框不参与统计" w265] -> w253
                        frame False {
                          # "取消 不把该框信息写入框组"
                          n146 = Delete From Array(array=w264) -> (array with subset deleted=w263:T3)  [unwired: 2 in, 1 out]
                        }
                        frame True {
                          # "0：位于蒙皮部位\n1：位于筋条部位"
                          # "存放部位信息的1D数组，后续生成报告使用"
                          n147 = Build Array(w276, w277) -> (w278:bool[])
                          n148 = Boolean Array To Number(Boolean array=w278) -> (number=w279:u32)
                          n149 = case shown="1, 默认" w279 {
                            tunnel: ["蒙皮处" ("t") "筋条处" ("t")] -> w267
                            frame 1, Default {
                            }
                            frame 2 {
                            }
                          }
                          n150 = local read "部位信息"() -> (w271:string[])
                          n151 = Decrement(x=w269) -> (x-1=w268:i32)
                          n152 = Insert Into Array(array=w271, index=w268, new element=w267) -> (w270:string[])
                          n153 = Concatenate Strings("框号为" ("字符串"), w272, "\n", "类别为" ("字符串"), w267) -> (w265:string)
                          n154 = local write "部位信息"(w270) -> ()
                        }
                      }
                      n155 = local write "连接的字符串"(w253) -> ()
                    }
                  }
                }
              }
              n156 = local read "完成标注"() -> (w203:bool)
              n157 = case shown="真" w203 {
                tunnel: [FALSE ("T button?") w210] -> w201
                frame False {
                }
                frame True {
                  n158 = Two Button Dialog(message="请确认是否完成标注\n完成标注后只能删除，无法新增标注" ("消息")) -> (T button?=w211:bool)  [unwired: 2 in]
                  n159 = case shown="真" w211 {
                    selector: w211 -> [_ w215]
                    tunnel: [FALSE w215] -> w210
                    frame False {
                    }
                    frame True {
                      w214 = T5."Enabled" ("禁用")
                      n160 = property on="导入图像" class="Bool"("DisabledEnum"=w214) -> ()  [unwired: 2 in, 2 out]
                      n161 = property on="删除标注" class="Bool (严格)"("DisabledEnum"=w214) -> ()  [unwired: 2 in, 2 out]
                      n162 = property on="查看评定结果" class="Bool (严格)"("DisabledEnum"=w214) -> ()  [unwired: 2 in, 2 out]
                      n163 = property on="生成报告" class="Bool"("DisabledEnum"=w214) -> ()  [unwired: 2 in, 2 out]
                    }
                  }
                }
              }
              n164 = local write "穿透图"(w206) -> ()
              n165 = local write "框组"(w198) -> ()
              n166 = local read "stop"() -> (w205:bool)
              n167 = Or(x=w205, y=w201) -> (x .or. y?=w197:bool)
              n168 = call <vilib>:"Application Directory.vi"() -> ()  [unwired: 1 out]
            }
          }
          frame 1 {
            # "对穿透图和反射图同时画框的分支"
            n169 = while {
              shift-right: [w285] -> _
              shift-left: T3 [] ("框组") -> [w294]
              tunnel: [w292] -> _
              tunnel: [w291] -> _
              stop <- w284 stop-if-true
              (unwired) "_" ("名称或相对路径")
              (unwired) ".docx" ("名称或相对路径")
              w290 = i32[] [2] items=["No Event"=0, "Click Event"=1, "Draw Event"=2, "Size Event"=4, "Scroll Event"=5, "Double Click Event"=8] ("Which Events")
              # "循环的方式给输入图像手动画框"
              n170 = local read "反射图"() -> (w293:T1)
              n171 = local read "穿透图"() -> (w287:T1)
              n172 = invoke on="穿透图" class="ImageControl" method="Get Last Event"("Which Events"=w290) -> ("Type"=w289:i32)  [unwired: 7 in, 7 out]
              n173 = Not Equal To 0?(x=w289) -> (x != 0?=w295:bool)
              n174 = case shown="真" w295 {
                tunnel: w287 -> [w306 w322]
                tunnel: [w306 w307] -> w292
                tunnel: [w305 w317] -> w285
                tunnel: w294 -> [w305 w321]
                tunnel: w293 -> [w304 w320]
                tunnel: [w304 w319] -> w291
                frame False {
                  n175 = Wait (ms)(milliseconds to wait=u32 50 ("毫秒倍数")) -> ()  [unwired: 1 out]
                }
                frame True {
                  n176 = property on="穿透图" class="ImageControl"() -> ("ROI"=w318:T6)  [unwired: 2 in, 2 out]
                  n177 = flat-sequence {
                    tunnel: w322 -> [w325]
                    tunnel: [w325] -> w316
                    tunnel: w318 -> [w327]
                    tunnel: [w327] -> w315
                    tunnel: w321 -> [w326]
                    tunnel: w320 -> [w324]
                    tunnel: [w324] -> w314
                    tunnel: [w323] -> w313
                    tunnel: w316 -> [w336]
                    tunnel: w315 -> [w335]
                    tunnel: w314 -> [w341]
                    tunnel: w313 -> [w328]
                    tunnel: [w342] -> w312
                    tunnel: [w340] -> w311
                    tunnel: [w328] -> w310
                    tunnel: [w332] -> w309
                    tunnel: [w330] -> w308
                    tunnel: w312 -> [w351]
                    tunnel: w311 -> [w359]
                    tunnel: w310 -> [w353]
                    tunnel: w309 -> [w355]
                    tunnel: w308 -> [w354]
                    tunnel: [w359] -> w319
                    tunnel: [w352] -> w317
                    tunnel: [w351] -> w307
                    frame #0 {
                      # "将当前ROI数据存入框组内"
                      n178 = Build Array (concatenate)(w326, w327) -> (w323:T3)
                    }
                    frame #1 {
                      w338 = u32[] [15663114] ("Colors (Green)")
                      w334 = u32 16711776 ("Text Color (black)")
                      # "在反射图上对应位置画框"
                      # "在穿透图上画框"
                      # "图层名Group与“框&图层计数”变量同名，\neg：1号框对应group1"
                      # "overlay text在ROI的左上角添加计数显示"
                      # "overlay ROI代表用户手画绿色框的图层添加"
                      n179 = Array Size(array=w328) -> (size(s)=w330:i32)
                      n180 = Unbundle(w335) -> ("Global Rectangle"=w347:i32[])  [unwired: 1 out]
                      n181 = Number To Decimal String(number=w330) -> (decimal integer string=w331:string)  [unwired: 1 in]
                      n182 = local write "框数"(w330) -> ()
                      n183 = Concatenate Strings(w331, "#" ("字符串")) -> (w332:string)
                      n184 = Index Array(array=w347, index=1 ("索引")) -> (element=w345:i32)
                      n185 = Index Array(array=w347, index=0 ("索引")) -> (element=w346:i32)
                      n186 = local read "自定义字体"() -> (w333:T2)
                      n187 = call "IMAQ Overlay ROI"("Colors (Green)"=w338, "Group"=w332, "ROI Descriptor"=w335, "Image"=w336) -> ("Image Out"=w348:T1)  [unwired: 6 in, 1 out]
                      n188 = call "IMAQ Overlay ROI"("Colors (Green)"=w338, "Group"=w332, "ROI Descriptor"=w335, "Image"=w341) -> ("Image Out"=w339:T1)  [unwired: 6 in, 1 out]
                      n189 = Bundle(w346, w345) -> (w337:cluster{i32, i32})  [unwired: 1 in]
                      n190 = call "IMAQ Overlay Text"("Group"=w332, "Text Color (black)"=w334, "Font, Size & Style"=w333, "String"=w332, "Origin"=w337, "Image"=w339) -> ("Image Out"=w340:T1)  [unwired: 4 in, 1 out]
                      n191 = call "IMAQ Overlay Text"("Group"=w332, "Text Color (black)"=w334, "Font, Size & Style"=w333, "String"=w332, "Origin"=w337, "Image"=w348) -> ("Image Out"=w342:T1)  [unwired: 4 in, 1 out]
                    }
                    frame #2 {
                      # "0：位于蒙皮部位\n1：位于筋条部位"
                      n192 = call "缺陷部位标注"() -> ("位于筋条处"=w357:bool, "位于蒙皮处"=w356:bool, "确定"=w349:bool)  [unwired: 16 in, 1 out]
                      n193 = Build Array(w356, w357) -> (w358:bool[])
                      n194 = case shown="真" w349 {
                        tunnel: w358 -> [_ w374]
                        tunnel: w355 -> [_ w370]
                        tunnel: w354 -> [_ w367]
                        tunnel: w353 -> [w362 w364]
                        tunnel: [w361 w364] -> w352
                        tunnel: ["由于点击取消，该框不参与统计" w363] -> w350
                        frame False {
                          # "取消 不把该框信息写入框组"
                          n195 = Delete From Array(array=w362) -> (array with subset deleted=w361:T3)  [unwired: 2 in, 1 out]
                        }
                        frame True {
                          # "存放部位信息的1D数组，后续生成报告使用"
                          n196 = Boolean Array To Number(Boolean array=w374) -> (number=w375:u32)
                          n197 = local read "部位信息"() -> (w369:string[])
                          n198 = case shown="1, 默认" w375 {
                            tunnel: ["蒙皮处" ("t") "筋条处" ("t")] -> w365
                            frame 1, Default {
                            }
                            frame 2 {
                            }
                          }
                          n199 = Decrement(x=w367) -> (x-1=w366:i32)
                          n200 = Insert Into Array(array=w369, index=w366, new element=w365) -> (w368:string[])
                          n201 = Concatenate Strings("框号为" ("字符串"), w370, "\n", "类别为" ("字符串"), w365) -> (w363:string)
                          n202 = local write "部位信息"(w368) -> ()
                        }
                      }
                      "连接的字符串" <- w350
                    }
                  }
                }
              }
              n203 = local read "完成标注"() -> (w283:bool)
              n204 = case shown="真" w283 {
                tunnel: [FALSE ("T button?") w297] -> w286
                frame False {
                }
                frame True {
                  n205 = Two Button Dialog(message="请确认是否完成标注\n完成标注后只能删除，无法新增标注" ("消息")) -> (T button?=w298:bool)  [unwired: 2 in]
                  n206 = case shown="真" w298 {
                    selector: w298 -> [_ w302]
                    tunnel: [FALSE w302] -> w297
                    frame False {
                    }
                    frame True {
                      w301 = T5."Enabled" ("禁用")
                      n207 = property on="生成报告" class="Bool"("DisabledEnum"=w301) -> ()  [unwired: 2 in, 2 out]
                      n208 = property on="删除标注" class="Bool (严格)"("DisabledEnum"=w301) -> ()  [unwired: 2 in, 2 out]
                      n209 = property on="查看评定结果" class="Bool (严格)"("DisabledEnum"=w301) -> ()  [unwired: 2 in, 2 out]
                      n210 = property on="导入图像" class="Bool"("DisabledEnum"=w301) -> ()  [unwired: 2 in, 2 out]
                    }
                  }
                }
              }
              n211 = local write "框组"(w285) -> ()
              n212 = local write "穿透图"(w292) -> ()
              n213 = local write "反射图"(w291) -> ()
              n214 = local read "stop"() -> (w288:bool)
              n215 = Or(x=w288, y=w286) -> (x .or. y?=w284:bool)
              n216 = call <vilib>:"Application Directory.vi"() -> ()  [unwired: 1 out]
            }
          }
        }
      }
      event "删除标注": Value Change {
        w379 = T5."Disabled and Grayed Out" ("禁用")
        n217 = event-data() -> ()  [unwired: 1 in, 6 out]
        n218 = call "用户输入2"() -> ("框号"=w380:dbl, "确定"=w381:bool)  [unwired: 17 in, 1 out]
        n219 = property on="生成报告" class="Bool"("DisabledEnum"=T5."Enabled" ("禁用")) -> ()  [unwired: 2 in, 2 out]
        n220 = property on="完成标注" class="Bool (严格)"("DisabledEnum"=w379) -> ()  [unwired: 2 in, 2 out]
        n221 = property on="开始标注" class="Bool"("DisabledEnum"=w379) -> ()  [unwired: 2 in, 2 out]
        n222 = case shown="真" w381 {
          tunnel: w380 -> [_ w382]
          frame False {
            # "用户取消操作"
          }
          frame True {
            n223 = stacked-sequence {
              tunnel: w382 -> [_ w389 _]
              frame #0 {
                # "1. 删除所有框"
                n224 = local read "穿透图"() -> (w383:T1)
                n225 = call "IMAQ Clear Overlay"("Image"=w383) -> ()  [unwired: 9 in, 2 out]
              }
              frame #1 {
                # "2. 删除框组中指定元素"
                n226 = local read "部位信息"() -> (w386:string[])
                n227 = local read "框组"() -> (w388:T3)
                n228 = Decrement(x=w389) -> (x-1=w385:dbl)
                n229 = Delete From Array(array=w386, index=w385) -> (array with subset deleted=w384:string[])  [unwired: 1 in, 1 out]
                n230 = Delete From Array(array=w388, index=w385) -> (array with subset deleted=w387:T3)  [unwired: 1 in, 1 out]
                n231 = local write "框组"(w387) -> ()
                n232 = local write "部位信息"(w384) -> ()
              }
              frame #2 {
                # "3. 重画所有框"
                n233 = while {
                  i -> [w402]
                  stop <- w393 stop-if-true
                  n234 = local read "框组"() -> (w397:T3)
                  n235 = local read "穿透图"() -> (w401:T1)
                  n236 = Array Size(array=w397) -> (size(s)=w398:i32)
                  n237 = Index Array(array=w397, index=w402) -> (element=w392:T6)
                  n238 = Increment(x=w402) -> (x+1=w409:i32)
                  n239 = local write "框数"(w398) -> ()
                  n240 = Greater Or Equal?(x=w409, y=w398) -> (x >= y?=w393:bool)
                  n241 = call "IMAQ Overlay ROI"("ROI Descriptor"=w392, "Image"=w401) -> ("Image Out"=w407:T1)  [unwired: 8 in, 1 out]
                  n242 = Unbundle(w392) -> ("Global Rectangle"=w399:i32[])  [unwired: 1 out]
                  n243 = Number To Decimal String(number=w409) -> (decimal integer string=w394:string)  [unwired: 1 in]
                  n244 = Index Array(array=w399, index=0 ("索引")) -> (element=w404:i32)
                  n245 = Index Array(array=w399, index=1 ("索引")) -> (element=w405:i32)
                  n246 = local read "自定义字体"() -> (w391:T2)
                  n247 = Concatenate Strings(w394, "#" ("字符串")) -> (w390:string)
                  n248 = Bundle(w404, w405) -> (w395:cluster{i32, i32})  [unwired: 1 in]
                  n249 = call "IMAQ Overlay Text"("Text Color (black)"=u32 16711680, "Font, Size & Style"=w391, "String"=w390, "Origin"=w395, "Image"=w407) -> ("Image Out"=w400:T1)  [unwired: 5 in, 1 out]
                  n250 = local write "穿透图"(w400) -> ()
                }
              }
            }
          }
        }
      }
      event "查看评定结果": Value Change {
        w413 = T5."Disabled and Grayed Out" ("禁用")
        # "只读穿透图的图像处理方法"
        # "查看指定框的详细信息，包括灰度和面积阈值分割后的结果，提取到的长宽面积等信息"
        n251 = event-data() -> ()  [unwired: 1 in, 6 out]
        n252 = property on="完成标注" class="Bool (严格)"("DisabledEnum"=w413) -> ()  [unwired: 2 in, 2 out]
        n253 = property on="开始标注" class="Bool"("DisabledEnum"=w413) -> ()  [unwired: 2 in, 2 out]
        n254 = local read "计入分层缺陷的面积阈值"() -> (w411:i32)
        n255 = local read "弥散类缺陷灰度阈值"() -> (w412:dbl)
        n256 = local read "分层类缺陷灰度阈值"() -> (w414:dbl)
        n257 = local read "临界面积百分比值"() -> (w416:dbl)
        n258 = local read "穿透图原始路径"() -> (w419:path)
        n259 = local read "临界Z值"() -> (w417:i32)
        n260 = local read "部位信息"() -> (w421:string[])
        n261 = local read "产品规格"() -> (w420:cluster{"产品长度（周长）（mm）":dbl, "产品宽度（母线长）（mm）":dbl})
        n262 = local read "框组"() -> (w418:T3)
        n263 = call "子VI-查看某框-读穿透图模式.vi"("输入框号（默认值0为整张图）"=0.0 ("框号"), "框组"=w418, "临界Z值"=w417, "弥散类缺陷灰度阈值"=w412, "临界面积百分比值"=w416, "分层缺陷的面积阈值"=w411, "预先配置的灰度阈值"=w414, "穿透图原始路径"=w419, "部位信息"=w421, "产品规格"=w420) -> ("全部检测结果"=→"全部检测结果":string[][])  [unwired: 17 in]
      }
      event "生成报告": Value Change {
        w426 = T5."Disabled and Grayed Out" ("禁用")
        # "相当于“查看标注”一栏中的操作做循环，遍历所有框，\n将输出结果叠加为数组，作为最终结果输出并导入word"
        n264 = event-data() -> ()  [unwired: 1 in, 6 out]
        n265 = call "报告模式选择"() -> ("深度学习方法"=w425:bool, "自动检测结果"=w428:bool, "手动框选结果"=w429:bool, "确定"=w427:bool)  [unwired: 15 in, 1 out]
        n266 = local read "计入分层缺陷的面积阈值"() -> (w422:i32)
        n267 = local read "分层类缺陷灰度阈值"() -> (w432:dbl)
        n268 = Build Array(w429, w428, w425) -> (w431:bool[])
        n269 = local read "临界面积百分比值"() -> (w433:dbl)
        n270 = local read "弥散类缺陷灰度阈值"() -> (w423:dbl)
        n271 = local read "穿透图原始路径"() -> (w436:path)
        n272 = Boolean Array To Number(Boolean array=w431) -> (number=w430:u32)
        n273 = local read "模式选择"() -> (w439:u16)
        n274 = local read "产品规格"() -> (w437:cluster{"产品长度（周长）（mm）":dbl, "产品宽度（母线长）（mm）":dbl})
        n275 = local read "部位信息"() -> (w438:string[])
        n276 = local read "框组"() -> (w435:T3)
        n277 = property on="删除标注" class="Bool (严格)"("DisabledEnum"=w426) -> ()  [unwired: 2 in, 2 out]
        n278 = property on="完成标注" class="Bool (严格)"("DisabledEnum"=w426) -> ()  [unwired: 2 in, 2 out]
        n279 = property on="开始标注" class="Bool"("DisabledEnum"=w426) -> ()  [unwired: 2 in, 2 out]
        n280 = local read "临界Z值"() -> (w434:i32)
        n281 = case shown="真" w427 {
          tunnel: w439 -> [_ w454]
          tunnel: w438 -> [_ w453]
          tunnel: w437 -> [_ w452]
          tunnel: w436 -> [_ w451]
          tunnel: w435 -> [_ w450]
          tunnel: w434 -> [_ w449]
          tunnel: w433 -> [_ w448]
          tunnel: string[][] [] ("分层类检测结果合并 2") -> [_ w447]
          tunnel: w432 -> [_ w446]
          tunnel: w430 -> [_ w445]
          tunnel: w423 -> [_ w442]
          tunnel: w422 -> [_ w441]
          frame False {
          }
          frame True {
            n282 = case shown="0, 默认" w445 {
              tunnel: [w464 w490 w520 w534] -> w455
              tunnel: w454 -> [_ _ _ _]
              tunnel: w453 -> [w467 w498 w527 _]
              tunnel: w452 -> [w466 w497 w526 w539]
              tunnel: w451 -> [w468 w496 w525 w538]
              tunnel: w450 -> [w469 w495 w524 _]
              tunnel: w449 -> [w471 w492 w523 w537]
              tunnel: w448 -> [w472 w493 w522 w536]
              tunnel: w447 -> [w473 w491 w519 w535]
              tunnel: w446 -> [w470 w494 w521 w531]
              tunnel: w442 -> [w462 w489 w518 w530]
              tunnel: w441 -> [w461 w488 w517 w529]
              frame 0, Default {
                # "只读穿透图的图像处理方法"
                # "默认手动框选结果"
                n283 = local read "框数"() -> (w465:dbl)
                n284 = for {
                  N: w465 -> [_]
                  shift-right: [w487] -> w464
                  shift-left: w473 -> [w486]
                  tunnel: w467 -> [w483]
                  tunnel: w466 -> [w482]
                  tunnel: w468 -> [w481]
                  tunnel: w469 -> [w480]
                  tunnel: w472 -> [w479]
                  tunnel: w470 -> [w478]
                  tunnel: w471 -> [w477]
                  tunnel: w462 -> [w475]
                  tunnel: w461 -> [w474]
                  i -> [w485]
                  n285 = Increment(x=w485) -> (x+1=w484:i32)
                  n286 = call "子VI-查看某框-不显示界面-只读穿透图模式.vi"("框号"=w484, "框组"=w480, "分层缺陷的面积阈值"=w474, "临界Z值"=w477, "弥散类缺陷灰度阈值"=w475, "临界面积百分比值"=w479, "预先配置的灰度阈值"=w478, "穿透图原始路径"=w481, "部位信息"=w483, "产品规格"=w482) -> ("全部检测结果"=w476:string[][])  [unwired: 17 in]
                  n287 = Build Array (concatenate)(w486, w476) -> (w487:string[][])
                }
                "报告模式" <- "手动框选"
              }
              frame 1 {
                # "只读穿透图的图像处理方法"
                n288 = local read "框数"() -> (w499:dbl)
                n289 = local write "报告模式"("手动框选") -> ()
                n290 = for {
                  N: w499 -> [_]
                  shift-right: [w514] -> w490
                  shift-left: w491 -> [w513]
                  tunnel: w498 -> [w510]
                  tunnel: w497 -> [w509]
                  tunnel: w496 -> [w508]
                  tunnel: w495 -> [w507]
                  tunnel: w494 -> [w506]
                  tunnel: w493 -> [w505]
                  tunnel: w492 -> [w504]
                  tunnel: w489 -> [w502]
                  tunnel: w488 -> [w501]
                  i -> [w512]
                  n291 = Increment(x=w512) -> (x+1=w511:i32)
                  n292 = call "子VI-查看某框-不显示界面-只读穿透图模式.vi"("框号"=w511, "框组"=w507, "分层缺陷的面积阈值"=w501, "临界Z值"=w504, "弥散类缺陷灰度阈值"=w502, "临界面积百分比值"=w505, "预先配置的灰度阈值"=w506, "穿透图原始路径"=w508, "部位信息"=w510, "产品规格"=w509) -> ("全部检测结果"=w503:string[][])  [unwired: 17 in]
                  n293 = Build Array (concatenate)(w513, w503) -> (w514:string[][])
                }
              }
              frame 2 {
                # "只读穿透图的图像处理方法"
                n294 = local write "报告模式"("自动检测") -> ()
                n295 = call "子VI-查看某框-不显示界面-只读穿透图模式.vi"("框号"=0.0, "框组"=w524, "分层缺陷的面积阈值"=w517, "临界Z值"=w523, "弥散类缺陷灰度阈值"=w518, "临界面积百分比值"=w522, "预先配置的灰度阈值"=w521, "穿透图原始路径"=w525, "部位信息"=w527, "产品规格"=w526) -> ("全部检测结果"=w515:string[][])  [unwired: 17 in]
                n296 = Build Array (concatenate)(w519, w515) -> (w520:string[][])
              }
              frame 4 {
                # "深度学习方法自动检测demo"
                n297 = local write "报告模式"("深度学习自动检测" ("报告模式")) -> ()
                n298 = call "子VI-深度学习自动检测.vi"("临界Z值"=w537, "弥散类缺陷灰度阈值"=w530, "临界面积百分比值"=w536, "分层缺陷的面积阈值"=w529, "产品规格"=w539, "穿透图原始路径"=w538, "输入的灰度阈值"=w531) -> ("全部检测结果"=w532:string[][])  [unwired: 8 in]
                n299 = Build Array (concatenate)(w532, w535) -> (w534:string[][])
              }
            }
            n300 = local write "全部检测结果合并"(w455) -> ()
            n301 = flat-sequence {
              tunnel: w455 -> [w540]
              tunnel: [w540] -> w460
              tunnel: w460 -> [w581]
              tunnel: [w581] -> w459
              tunnel: w459 -> [w587]
              tunnel: [w587] -> w458
              tunnel: [w583] -> w444
              tunnel: [w582] -> w443
              tunnel: [w614] -> w457
              tunnel: [w613] -> w456
              tunnel: w458 -> [w607]
              tunnel: w444 -> [w604]
              tunnel: w443 -> [w603]
              tunnel: w456 -> [w633]
              tunnel: w457 -> [w634]
              frame #0 {
                n302 = while {
                  tunnel: [w558] -> _
                  i -> [w560]
                  stop <- w558 stop-if-true
                  w565 = 1 items=["White", "Black", "Inverted", "Black on White", "White on Black"] ("Color")
                  w567 = u16 2 items=["Frame", "Paint", "Invert Frame", "Invert Paint"] ("Draw Mode")
                  w562 = u16 1 items=["Line", "Rectangle", "Oval"] ("Shape to draw")
                  # "生成绘制了ROI的图像\n可以用于后续的图片导出保存"
                  n303 = local read "框组"() -> (w559:T3)
                  n304 = local read "ROImask"() -> (w555:T1)
                  n305 = local read "穿透图"() -> (w556:T1)
                  n306 = Array Size(array=w559) -> (size(s)=w568:i32)
                  n307 = Index Array(array=w559, index=w560) -> (element=w553:T6)
                  n308 = Unbundle By Name(w553) -> ("Global Rectangle"=w548:i32[])
                  n309 = Increment(x=w560) -> (x+1=w569:i32)
                  n310 = Greater Or Equal?(x=w569, y=w568) -> (x >= y?=w558:bool)
                  n311 = Index Array(array=w548, index=2 ("索引")) -> (element=w547:i32)
                  n312 = Index Array(array=w548, index=0 ("索引")) -> (element=w544:i32)
                  n313 = Index Array(array=w548, index=3 ("索引")) -> (element=w546:i32)
                  n314 = Index Array(array=w548, index=1 ("索引")) -> (element=w543:i32)
                  n315 = Number To Decimal String(number=w569) -> (decimal integer string=w563:string)  [unwired: 1 in]
                  n316 = Build Array(w544, w543, w547, w546) -> (w545:i32[])
                  n317 = call "IMAQ Draw"("Draw Mode"=w567, "Shape to draw"=w562, "Coordinates"=w545, "Image Src"=w556) -> ("Image Dst Out"=w566:T1)  [unwired: 6 in, 1 out]
                  n318 = Concatenate Strings(w563, "#" ("字符串")) -> (w561:string)
                  n319 = local read "自定义字体"() -> (w557:T2)
                  n320 = Build Array(w544, w543) -> (w542:i32[])
                  n321 = call "IMAQ Draw Text"("String"=w561, "Insertion Point"=w542, "Color"=w565, "Font, Size & Style"=w557, "Image Dst"=w555, "Image Src"=w566) -> ("error out"=w541:errorcluster, "Image Dst Out"=w554:T1)  [unwired: 2 in, 2 out]
                  "ROImask" <- w554
                  n322 = case shown="错误" w541 {
                    frame No Error {
                    }
                    frame Error {
                      n323 = One Button Dialog(message="失败！无法保存图片到报告" ("消息")) -> ()  [unwired: 1 in, 1 out]
                    }
                  }
                  n324 = local write "ROImask"(w554) -> ()
                }
              }
              frame #1 {
                n325 = local read "穿透图原始路径"() -> (w580:path)
                n326 = local read "ROImask"() -> (w572:T1)
                n327 = Path To String(path=w580) -> (string=w577:string)
                n328 = String Length(string=w577) -> (length=w578:i32)
                n329 = Subtract(x=w578, y=4) -> (x-y=w579:i32)
                n330 = Replace Substring(3:w579, 4:"_标注后.png" ("字符串"), 5:w577) -> (1:w576:string)  [unwired: 1 in, 1 out]
                n331 = String To Path(string=w576) -> (path=w571:path)
                "标注后的图片路径" <- w571
                n332 = call-poly "IMAQ Write File 2"("Image Quality"=u32 1000, "File Path"=w571, "Image"=w572) -> ()  [unwired: 7 in, 2 out]
              }
              frame #2 {
                # "最终检测结果全部合并 导入word中"
                n333 = call <vilib>:"Application Directory.vi"() -> ("Application Directory"=w586:path)
                n334 = Build Path(base path=w586, name or relative path="report-template.docx") -> (appended path=w584:path)
                n335 = call <vilib>:"Create Report.vi"("window state (normal)"=T8."maximized", "report type"=Report_Type."Word", "template (empty)"=w584) -> ("report out"=w583:refnum<class "NI_report.lvclass">, "error out"=w582:errorcluster)  [unwired: 11 in]
              }
              frame #3 {
                n336 = local read "报告模式"() -> (w605:string)
                n337 = local read "质量等级"() -> (w601:string)
                n338 = local read "标注后的图片路径"() -> (w594:path)
                n339 = Get Date/Time String(date format (0)=enum16{"short", "long", "abbreviated"}."long" ("日期格式(0)")) -> (date string=w611:string, time string=w612:string)  [unwired: 2 in]
                n340 = call-poly <vilib>:"Append Report Text.vi"("report in"=w604, "MS Office parameters"=T12 {"position (excel)"={"row"=0, "column"=0}, "name (excel)"="", "bookmark (word)"="mode"}, "text"=w605, "error in (no error)"=w603) -> ("report out"=w600:refnum<class "NI_report.lvclass">, "error out"=w599:errorcluster)  [unwired: 8 in, 2 out]
                n341 = Concatenate Strings(w611, w612) -> (w610:string)
                n342 = call-poly <vilib>:"Append Report Text.vi"("report in"=w600, "MS Office parameters"=T12 {"position (excel)"={"row"=0, "column"=0}, "name (excel)"="", "bookmark (word)"="class"}, "text"=w601, "error in (no error)"=w599) -> ("report out"=w597:refnum<class "NI_report.lvclass">, "error out"=w598:errorcluster)  [unwired: 8 in, 2 out]
                n343 = call-poly <vilib>:"Append Report Text.vi"("report in"=w597, "MS Office parameters"=T12 {"position (excel)"={"row"=0, "column"=0}, "name (excel)"="", "bookmark (word)"="time"}, "text"=w610, "error in (no error)"=w598) -> ("report out"=w592:refnum<class "NI_report.lvclass">, "error out"=w591:errorcluster)  [unwired: 8 in, 2 out]
                n344 = call-poly <vilib>:"Append Image to Report.vi"("report in"=w592, "alignment (default)"=HTML_Report_Image_Alignment."MIDDLE", "MS Office parameters"=T11 {"position (Excel)"={"row"=0, "column"=0}, "name (Excel)"="", "bookmark (Word)"="image"}, "path or URL of image"=w594) -> ("report out"=w590:refnum<class "NI_report.lvclass">, "error out"=w593:errorcluster)  [unwired: 8 in, 2 out]
                n345 = call <vilib>:"Word Easy Text.vi"("report in"=w590, "text"="检测结果：", "alignment (left)"=enum16{"Left", "Centered", "Right", "Justify"}."Left", "font"=T13 {"font name"="", "font size"=0.0, "bold"=0, "italic"=0, "underline"=0, "strike through"=0, "font color"=16777216}, "error in (no error)"=w591) -> ("report out"=w616:refnum<class "NI_report.lvclass">, "error out"=w617:errorcluster)  [unwired: 8 in, 1 out]
                n346 = case shown="错误" w593 {
                  frame No Error {
                  }
                  frame Error {
                    n347 = One Button Dialog(message="图片导入word\n发生错误！" ("消息")) -> ()  [unwired: 1 in, 1 out]
                  }
                }
                n348 = call-poly <vilib>:"Word Easy Table.vi"("report in"=w616, "column headers"=string[] ["框号", "X/mm", "Y/mm", "长/mm", "宽/mm", "面积/mm2", "Z值/mm", "部位", "类型", "合格性"], "data"=w607, "error in (no error)"=w617) -> ("report out"=w614:refnum<class "NI_report.lvclass">, "error out"=w613:errorcluster)  [unwired: 9 in, 1 out]
              }
              frame #4 {
                n349 = local read "穿透图原始路径"() -> (w626:path)
                n350 = local read "报告模式"() -> (w624:string)
                n351 = Path To String(path=w626) -> (string=w630:string)
                n352 = String Length(string=w630) -> (length=w631:i32)
                n353 = Subtract(x=w631, y=4) -> (x-y=w632:i32)
                n354 = Concatenate Strings("_" ("字符串"), w624, "_.docx" ("字符串")) -> (w622:string)
                n355 = Replace Substring(3:w632, 4:w622, 5:w630) -> (1:w629:string)  [unwired: 1 in, 1 out]
                n356 = String To Path(string=w629) -> (path=w627:path)
                "添加的路径" <- w627
                n357 = call-dynamic "Save Report to File.vi"("report in"=w634, "report file path"=w627, "prompt to replace? (F)"=TRUE, "error in (no error)"=w633) -> ("report out"=w638:refnum<class "NI_report.lvclass">, "error out"=w637:errorcluster)  [unwired: 10 in]
                n358 = call <vilib>:"Word Bring to Front.vi"("report in"=w638, "window state (maximized)"=enum16{"maximized", "minimized", "normal"}."normal", "error in (no error)"=w637) -> ()  [unwired: 11 in, 2 out]
              }
              frame #5 {
                n359 = local write "全部检测结果合并"(string[][] [] ("弥散类检测结果合并")) -> ()
                n360 = One Button Dialog(message="完成评定并退出程序！\n请查看word报告" ("消息")) -> ()  [unwired: 1 in, 1 out]
              }
            }
          }
        }
      }
      event "stop": Value Change {
        # "退出软件"
        n361 = event-data() -> ("NewVal"=w644:bool)  [unwired: 1 in, 4 out]
        n362 = Two Button Dialog(message="是否关闭本软件？" ("消息")) -> (T button?=w645:bool)  [unwired: 2 in]
        n363 = And(x=w644, y=w645) -> (x .and. y?=w643:bool)
        n364 = case shown="真" w643 {
          frame False {
          }
          frame True {
            w646 = TRUE ("All Images? (No)")
            n365 = local read "穿透图"() -> (w648:T1)
            n366 = local read "反射图"() -> (w647:T1)
            n367 = call "IMAQ Dispose"("All Images? (No)"=w646, "Image"=w648) -> ()  [unwired: 4 in, 1 out]
            n368 = call "IMAQ Dispose"("All Images? (No)"=w646, "Image"=w647) -> ()  [unwired: 4 in, 1 out]
            n369 = disable-structure shown="RUN_TIME_ENGINE==True" {
              frame condition #0 {
                n370 = Quit LabVIEW() -> ()  [unwired: 1 in]
              }
              frame condition #1 (active) {
                n371 = Stop() -> ()  [unwired: 1 in]
              }
            }
          }
        }
      }
    }
  }
  n372 = disable-structure shown="禁用" {
    frame Disabled {
      n373 = while {
        stop <- FALSE stop-if-true
        n374 = local read "查看评定结果"() -> (w651:bool)
        n375 = local read "删除标注"() -> (w652:bool)
        n376 = Or(x=w652, y=w651) -> (x .or. y?=w653:bool)
        n377 = local write "开始标注"(w653) -> ()
        n378 = Wait Until Next ms Multiple(millisecond multiple=u32 50 ("毫秒倍数")) -> ()  [unwired: 1 out]
      }
    }
    frame Enabled {
    }
  }
  n379 = disable-structure shown="禁用" {
    frame Disabled {
    }
    frame Enabled {
    }
  }
  "临界面积百分比值" <- w10
  "分层类缺陷灰度阈值" <- w11
  "弥散类缺陷灰度阈值" <- w1
